vi "Obtain UI-RT Stream Endpoints.vi"(8 "New":bool, 9 "Connect Timeout(ms) in":i32, 10 "reader endpoint":refnum<k21>, 11 "writer endpoint":refnum<k21>) -> (1 "Connect Timeout(ms)":i32, 2 "UI Command Stream":refnum<k21>, 3 "RT Message Stream":refnum<k21>)   [LabVIEW 2015, in "Tool Interface.lvlib"]
uses:
  Tool Interface.lvlib
  Tool Typedefs/Message Cluster.ctl
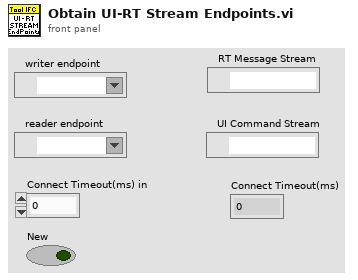
[diagram p1: front panel]
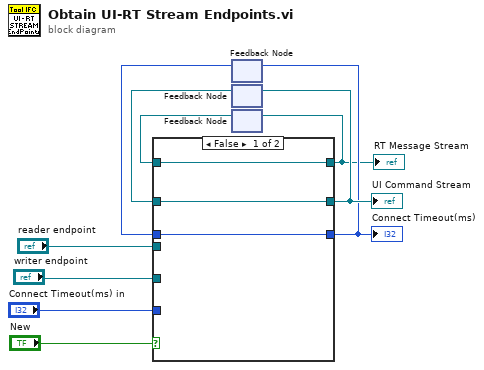
[diagram p0: block diagram]
diagram:
  n1 = feedback #1() -> (w4:i32)  [unwired: 1 in]
  n2 = feedback #2() -> (w7:refnum<k21>)  [unwired: 1 in]
  n3 = feedback #3() -> (w9:refnum<k21>)  [unwired: 1 in]
  n4 = case shown="False" "New" {
    tunnel: "reader endpoint" -> [_ w16]
    tunnel: "writer endpoint" -> [_ w15]
    tunnel: [w13 w16] -> w1
    tunnel: [w12 w15] -> w8
    tunnel: w9 -> [w13 _]
    tunnel: w7 -> [w12 _]
    tunnel: [w11 w14] -> w5
    tunnel: "Connect Timeout(ms) in" -> [_ w14]
    tunnel: w4 -> [w11 _]
    frame False {
    }
    frame True {
    }
  }
  "Connect Timeout(ms)" <- w5
  "RT Message Stream" <- w1
  "UI Command Stream" <- w8
  n5 = feedback-in #1(w5) -> ()
  n6 = feedback-in #2(w8) -> ()
  n7 = feedback-in #3(w1) -> ()
